vi "Write Configuration.vi"(8 "error in (no error)":errorcluster, 10 "Variant":variant, 11 "Configuration in":refnum<class "Configuration.lvclass">) -> (0 "error out":errorcluster, 3 "Configuration out":refnum<class "Configuration.lvclass">)   [LabVIEW 2016, in "Configuration.lvclass"]
uses:
  Configuration.lvclass
  Configuration.lvclass/Configuration.ctl
  <vilib>/Utility/config.llb/NI_LVConfig.lvlib
  <vilib>/addons/_JKI.lib/Serialization/JSON/JKI JSON Serialization.lvlib
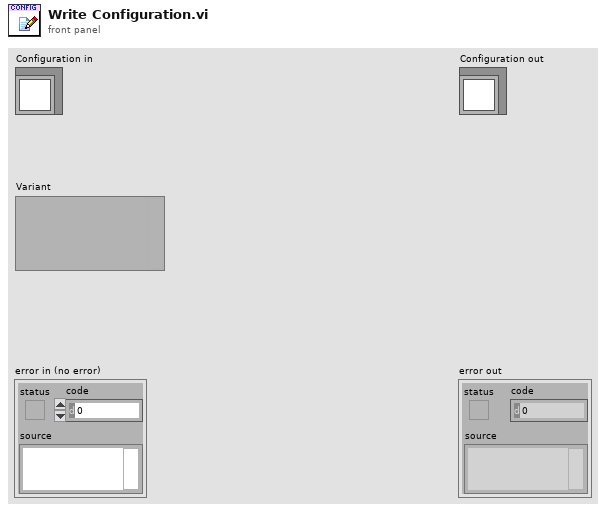
[diagram p1: front panel]
types:
  T1 = typedef "NI_LVConfig.lvlib/Config Data RefNum.ctl" = refnum<k1>
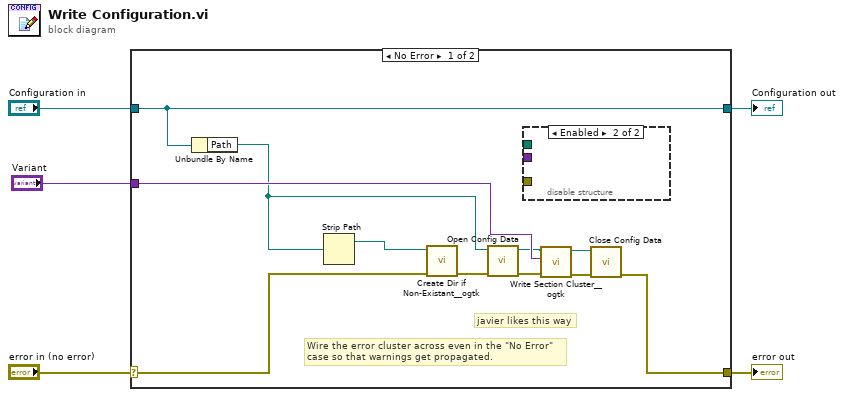
[diagram p0: block diagram]
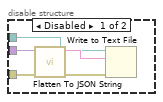
[diagram p2: hidden frame]
diagram:
  n1 = case shown="No Error" "error in (no error)" {
    selector: "error in (no error)" -> [w7 w23]
    tunnel: [w10 w23] -> w4
    tunnel: [w16 w22] -> w2
    tunnel: "Configuration in" -> [w16 w22]
    tunnel: "Variant" -> [w15 _]
    frame No Error {
      # "javier likes this way"
      # "Wire the error cluster across even in the \"No Error\"\ncase so that warnings get propagated."
      n2 = Unbundle By Name(w16) -> ("Path"=w8:path)
      n3 = Strip Path(path=w8) -> (stripped path=w6:path)  [unwired: 1 out]
      n4 = call <userlib>:"Create Dir if Non-Existant__ogtk.vi"("error in (no error)"=w7, "Directory Path"=w6) -> ("error out"=w9:errorcluster)  [unwired: 7 in, 2 out]
      n5 = call <vilib>:"Open Config Data.vi"("error in (no error)"=w9, "configuration file path"=w8) -> ("error out"=w14:errorcluster, "refnum"=w13:T1)  [unwired: 7 in, 1 out]
      n6 = disable-structure shown="Enabled" {
        disable-tunnel: _ -> [w21 _]
        disable-tunnel: _ -> [w20 _]
        disable-tunnel: _ -> [w17 _]
        frame Disabled {
          n7 = call <vilib>:"Flatten To JSON String.vi"("error in (no error)"=w21, "Variant"=w20) -> ("error out"=w19:errorcluster, "JSON String"=w18:string)  [unwired: 8 in]
          n8 = Write to Text File(file (use dialog)=w17, text=w18, error in=w19) -> ()  [unwired: 1 in, 3 out]
        }
        frame Enabled {
        }
      }
      n9 = call <userlib>:"Write Section Cluster__ogtk.vi"("error in (no error)"=w14, "Section Formatted Cluster"=w15, "refnum"=w13) -> ("error out"=w12:errorcluster, "dup refnum"=w11:T1)  [unwired: 7 in]
      n10 = call <vilib>:"Close Config Data.vi"("error in (no error)"=w12, "refnum"=w11) -> ("error out"=w10:errorcluster)  [unwired: 8 in, 1 out]
    }
    frame Error {
    }
  }
  "error out" <- w4
  "Configuration out" <- w2
